vi "Singles_Doubles.vi"(11 "Name":string) -> (0 "AllLetters":string[](array[string]), 3 "Singles&Doubles":string[](array[string]))   [LabVIEW 2014]
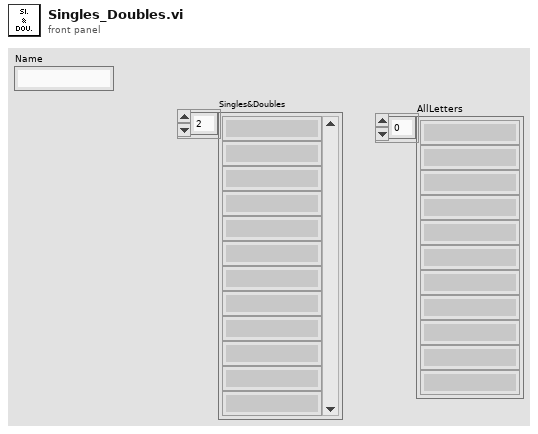
[diagram p1: front panel]
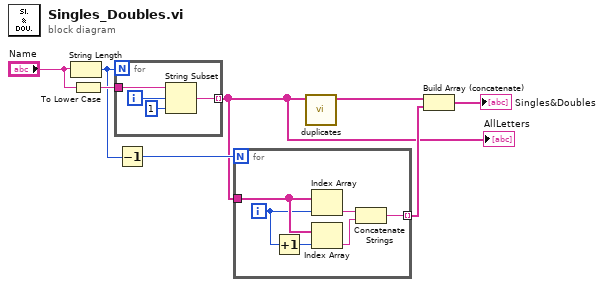
[diagram p0: block diagram]
diagram:
  n1 = String Length(string="Name") -> (length=w5:i32)
  n2 = To Lower Case(string="Name") -> (all lower case string=w6:string)
  n3 = for {
    N: w5 -> [_]
    tunnel: [w10] -> w2 mode=indexing
    tunnel: w6 -> [w9]
    i -> [w11]
    n4 = String Subset(string=w9, offset (0)=w11, length (rest)=1 ("length (rest)")) -> (substring=w10:string)
  }
  "AllLetters" <- w2
  n5 = Decrement(x=w5) -> (x-1=w8:i32)
  n6 = for {
    N: w8 -> [_]
    tunnel: w2 -> [w18]
    tunnel: [w13] -> w7 mode=indexing
    i -> [w16]
    n7 = Increment(x=w16) -> (x+1=w17:i32)
    n8 = Index Array(array=w18, index=w16) -> (element=w15:string)
    n9 = Index Array(array=w18, index=w17) -> (element=w14:string)
    n10 = Concatenate Strings(w15, w14) -> (w13:string)
  }
  n11 = call "duplicates.vi"("Array"=w2) -> ("Array 2"=w3:string[])  [unwired: 10 in]
  n12 = Build Array (concatenate)(w3, w7) -> (→"Singles&Doubles":string[])
